vi "HandShake.vi"(8 "error in (no error)":errorcluster, 10 "Data In":u8[](array[numeric]), 11 "InferenceTCP in":refnum<class "InferenceTCP.lvclass">) -> (0 "error out":errorcluster, 2 "Data Out":string, 3 "InferenceTCP out":refnum<class "InferenceTCP.lvclass">)   [LabVIEW 2021, in "InferenceTCP.lvlib" / "InferenceTCP.lvclass"]
uses:
  InferenceTCP.lvclass
  InferenceTCP.lvclass/InferenceTCP.ctl
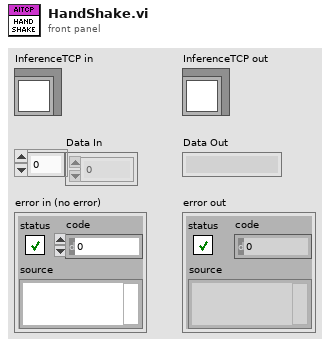
[diagram p1: front panel]
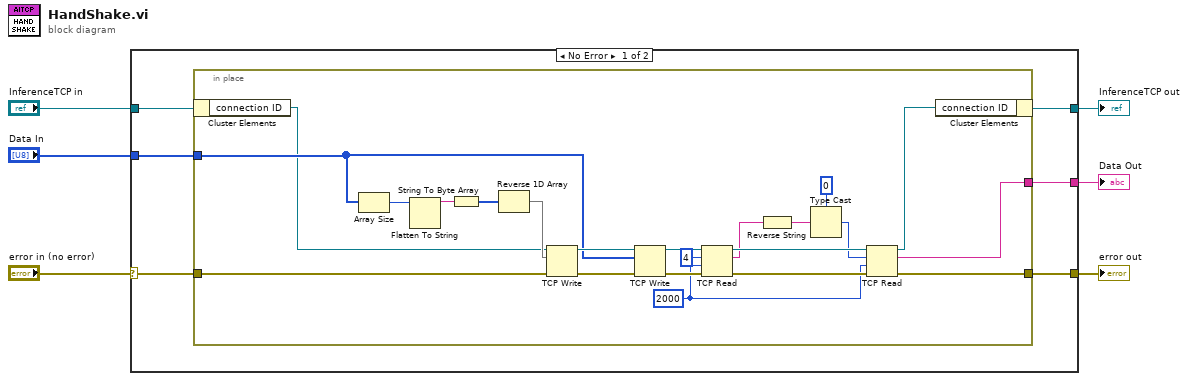
[diagram p0: block diagram]
diagram:
  n1 = case shown="No Error" "error in (no error)" {
    selector: "error in (no error)" -> [w8 w36]
    tunnel: [w7 w36] -> w5
    tunnel: [w10 w35] -> w3
    tunnel: "InferenceTCP in" -> [w12 w35]
    tunnel: "Data In" -> [w11 _]
    tunnel: [w9 _] -> w1
    frame No Error {
      n2 = in-place {
        in-place-border: w11 -> [w19]
        in-place-border: [w16] -> w9
        in-place-border: w8 -> [w15]
        in-place-border: [w14] -> w7
        w13 = 2000 ("timeout ms (25000)")
        n3 = in-place-cluster #1(w12) -> ("connection ID"=w18:refnum<k5>)
        n4 = Array Size(array=w19) -> (size(s)=w32:i32)
        n5 = Flatten To String(anything=w32) -> (data string=w34:string)  [unwired: 3 in, 2 out]
        n6 = String To Byte Array(string=w34) -> (unsigned byte array=w33:u8[])
        n7 = Reverse 1D Array(array=w33) -> (reversed array=w31:u8[])
        n8 = TCP Write(connection ID=w18, data in=w31, error in (no error)=w15) -> (connection ID out=w30:refnum<k5>, error out=w29:errorcluster)  [unwired: 1 in, 1 out]
        n9 = TCP Write(connection ID=w30, data in=w19, error in (no error)=w29) -> (connection ID out=w28:refnum<k5>, error out=w27:errorcluster)  [unwired: 1 in, 1 out]
        n10 = TCP Read(connection ID=w28, bytes to read=4, error in (no error)=w27, 9:w13) -> (connection ID out=w26:refnum<k5>, data out=w23:string, error out=w25:errorcluster)  [unwired: 1 in]
        n11 = Reverse String(1:w23) -> (0:w20:string)
        n12 = Type Cast(type=0 ("bytes to read"), x=w20) -> (*(type *) &x=w21:i32)
        n13 = TCP Read(connection ID=w26, bytes to read=w21, error in (no error)=w25, 9:w13) -> (connection ID out=w17:refnum<k5>, data out=w16:string, error out=w14:errorcluster)  [unwired: 1 in]
        n14 = in-place-cluster #1("connection ID"=w17) -> (w10:refnum<class "InferenceTCP.lvclass">)
      }
    }
    frame Error {
    }
  }
  "error out" <- w5
  "InferenceTCP out" <- w3
  "Data Out" <- w1
